vi "MPB_enqueue test results.vi"(8 "error in":errorcluster, 10 "test results":T1={"test pass"=FALSE, "step_type"=enum."prompt", "value"=0.0, "step description"="", "error"={"status"=FALSE, "code"=0, "source"=""}, "save results"=FALSE}, 11 "queue in":refnum<queue>) -> (0 "error out":errorcluster, 3 "queue out":refnum<queue>)   [LabVIEW 2020]
uses:
  controls/test results.ctl
  controls/MPB_step_type.ctl
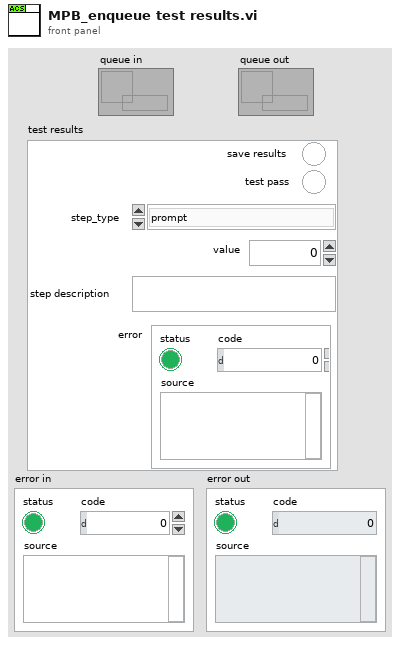
[diagram p1: front panel]
types:
  T1 = typedef "test results.ctl" = cluster{"test pass":bool, "step_type":T2, "value":dbl, "step description":string, "error":errorcluster, "save results":bool}
  T2 = typedef "MPB_step_type.ctl" = enum16{"default", "prompt", "sequence#", "12V_1_power supply on_off", "12V_2_power supply on_off", "set_hipot_V", "set_hipot_I_limit", "set_hipot_ramping (sec)", "set hipot_hold_time", "read_hipot_V", "read_hipot_I", "set_daq", "read_daq", "flash uds", "wait (sec)", "record_pass_fail", "ac_charge_test", "dc_400V_charging", "HAPS Heater Output", "HAPS Compressor Output", "stop_test", "error_exit"}
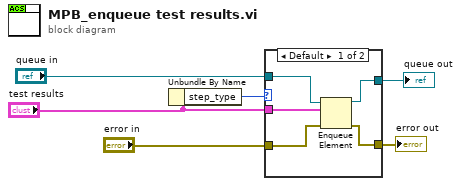
[diagram p0: block diagram]
diagram:
  n1 = Unbundle By Name("test results") -> ("step_type"=w4:T2)
  n2 = case shown="Default" w4 {
    tunnel: "error in" -> [w11 w12]
    tunnel: [w10 w12] -> w5
    tunnel: "queue in" -> [w9 w13]
    tunnel: [w8 w13] -> w1
    tunnel: "test results" -> [w7 _]
    frame Default {
      n3 = Enqueue Element(queue=w9, element=w7, error in (no error)=w11) -> (queue out=w8:refnum<queue>, error out=w10:errorcluster)  [unwired: 1 in, 1 out]
    }
    frame "default" {
    }
  }
  "error out" <- w5
  "queue out" <- w1
